vi "Actor Core.vi"(8 "error in":errorcluster, 11 "Vacuum in":refnum<class "Vacuum.lvclass">) -> (0 "error out":errorcluster, 3 "Actor out":refnum<class "Actor.lvclass">)   [LabVIEW 2015, in "AMS UI.lvlib" / "Vacuum.lvclass"]
doc: "(<B>Filename</B>: Actor Framework.lvlib:Actor.lvclass:Actor Core.vi)\n\nReceives messages to the actor, reacts to them, and initiates any error handling that may shut the actor down.\n\nDescendant classes may override this VI to append parallel tasks for the actor to complete while it handles messages. Overrides use the Call Parent Method node."
uses:
  Vacuum.lvclass
  <vilib>/ActorFramework/Actor/Actor.lvclass
  <vilib>/ActorFramework/Actor/Actor.lvclass/Actor.ctl
  <vilib>/ActorFramework/Message Enqueuer/Message Enqueuer.lvclass/Message Enqueuer.ctl
  <vilib>/ActorFramework/Message Enqueuer/Init from Existing Queue.vi
  AMS Gas Actor/AMS Gas Actor.lvclass
  <vilib>/ActorFramework/Message Enqueuer/Message Enqueuer.lvclass
  eActor/eActor.lvclass
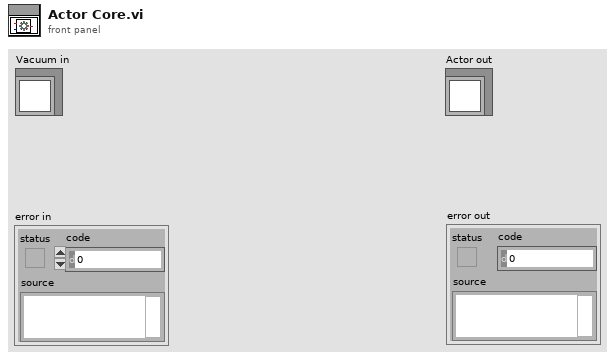
[diagram p1: front panel]
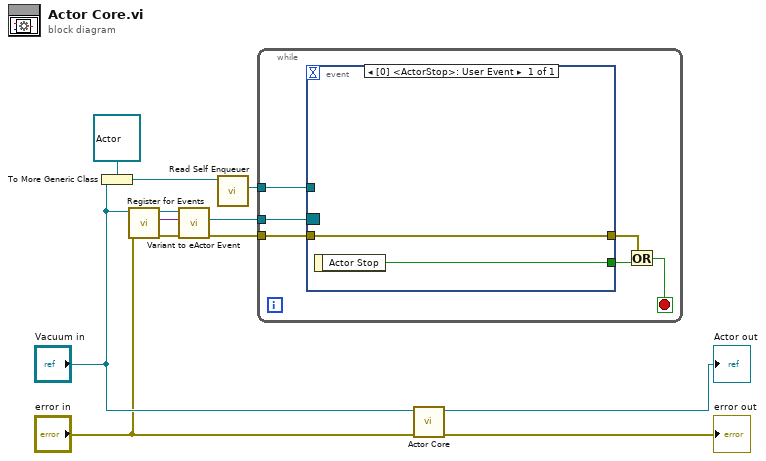
[diagram p0: block diagram]
diagram:
  n1 = To More Generic Class(target class=refnum<class "Actor.lvclass"> refnum ("Actor"), reference="Vacuum in") -> (generic class reference=w8:refnum<class "Actor.lvclass">)
  n2 = call-dynamic "Register for Events.vi"("error in (no error)"="error in", "eActor in"="Vacuum in") -> ("error out"=w2:errorcluster, "Event Registration Refnum"=w11:variant, "eActor out"=w3:refnum<class "Vacuum.lvclass">)  [unwired: 7 in]
  n3 = call "Variant to eActor Event.vi"("error in (no error)"=w2, "Variant"=w11, "eActor in"=w3) -> ("error out"=w1:errorcluster, "Event Registration Refnum"=w4:refnum<event-registration>)  [unwired: 6 in, 1 out]
  n4 = call <vilib>:"Read Self Enqueuer.vi"("Actor"=w8) -> ("Self Enqueuer"=w10:refnum<class "Message Enqueuer.lvclass">)  [unwired: 10 in]
  n5 = while {
    tunnel: w1 -> [w17]
    tunnel: w4 -> [w18]
    tunnel: w10 -> [w16]
    stop <- w15 stop-if-true
    n6 = event shown="[0] <ActorStop>: User Event" {
      selector: w18 -> [_]
      dyn-events: _ -> [_]
      timeout: _ -> [_]
      tunnel: w17 -> [w20]
      tunnel: [w19] -> w13
      tunnel: w16 -> [_]
      tunnel: [w20] -> w14
      event User Event {
        n7 = event-data() -> ("Actor Stop"=w19:bool)  [unwired: 1 in]
      }
    }
    n8 = Or(x=w14, y=w13) -> (x .or. y?=w15:bool)
  }
  n9 = call-parent "Actor Core.vi"("error in"="error in", "Actor in"="Vacuum in") -> ("error out"=→"error out":errorcluster, "Actor out"=→"Actor out":refnum<class "Actor.lvclass">)  [unwired: 8 in]
